vi "WriteGPSRefernceData.vi"(0 "LatitudeRef":string="South", 1 "ExifTool Path":path=path "C:/Windows/System32", 5 "LongitudeRef":string="East", 7 "AltitudeRef":string="Above Sea Level", 9 "filepath":string, 11 "error in (no error)":errorcluster, 12 "wait until completion? (T)":bool=TRUE) -> (4 "standard error":string, 15 "error out":errorcluster)   [LabVIEW 2016]
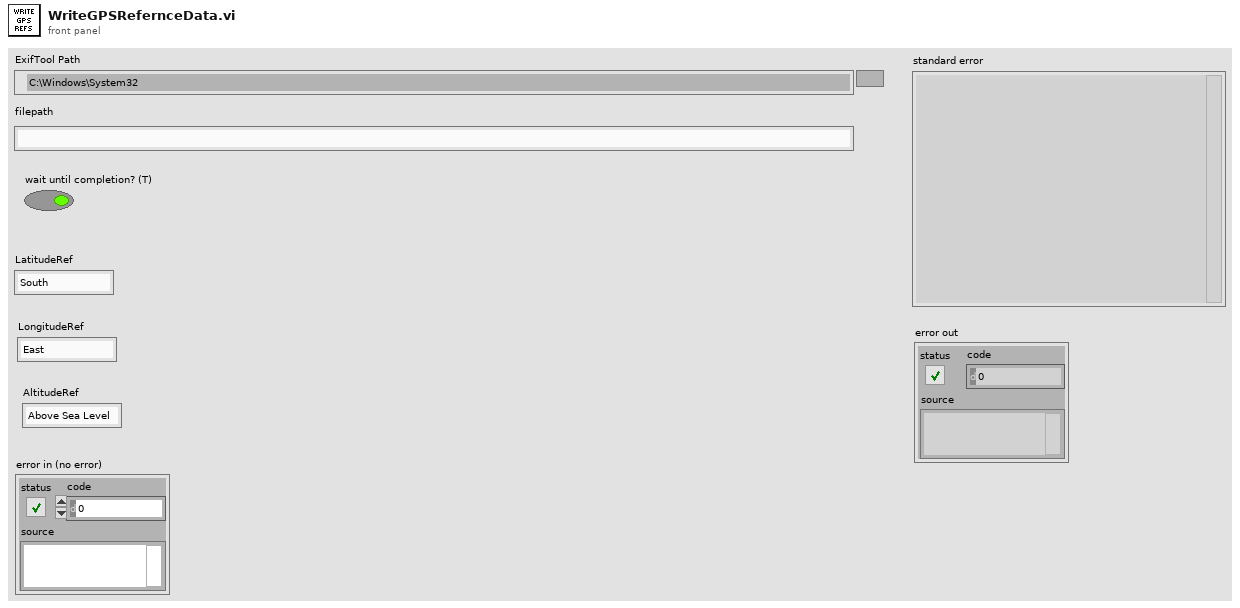
[diagram p1: front panel]
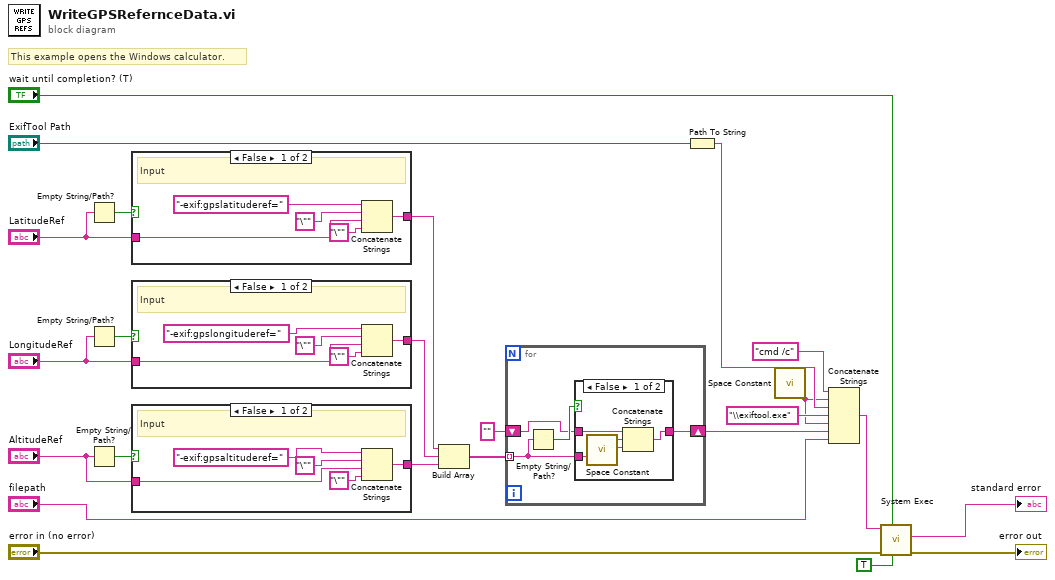
[diagram p0: block diagram]
diagram:
  # "This example opens the Windows calculator."
  n1 = Empty String/Path?(string/path="LatitudeRef") -> (empty?=w18:bool)
  n2 = Empty String/Path?(string/path="LongitudeRef") -> (empty?=w15:bool)
  n3 = Empty String/Path?(string/path="AltitudeRef") -> (empty?=w13:bool)
  n4 = case shown="False" w18 {
    tunnel: "LatitudeRef" -> [w27 _]
    tunnel: [w25 _] -> w12
    frame False {
      # "Input"
      n5 = Concatenate Strings("-exif:gpslatituderef=" ("string"), "\"" ("string"), w27, "\"" ("string")) -> (w25:string)
    }
    frame True {
    }
  }
  n6 = case shown="False" w15 {
    tunnel: "LongitudeRef" -> [w32 _]
    tunnel: [w30 _] -> w11
    frame False {
      # "Input"
      n7 = Concatenate Strings("-exif:gpslongituderef=" ("string"), "\"" ("string"), w32, "\"" ("string")) -> (w30:string)
    }
    frame True {
    }
  }
  n8 = case shown="False" w13 {
    tunnel: "AltitudeRef" -> [w37 _]
    tunnel: [w35 _] -> w10
    frame False {
      # "Input"
      n9 = Concatenate Strings("-exif:gpsaltituderef=" ("string"), "\"" ("string"), w37, "\"" ("string")) -> (w35:string)
    }
    frame True {
    }
  }
  n10 = Build Array(w12, w11, w10) -> (w9:string[])
  n11 = for {
    tunnel: w9 -> [w40] mode=indexing
    shift-right: [w41] -> w7
    shift-left: "" -> [w42]
    n12 = Empty String/Path?(string/path=w40) -> (empty?=w43:bool)
    n13 = case shown="False" w43 {
      tunnel: w42 -> [w47 w48]
      tunnel: [w45 w48] -> w41
      tunnel: w40 -> [w44 _]
      frame False {
        n14 = call <vilib>:"Space Constant.vi"() -> ("String"=w46:string)
        n15 = Concatenate Strings(w47, w44, w46) -> (w45:string)
      }
      frame True {
      }
    }
  }
  n16 = Path To String(path="ExifTool Path") -> (string=w21:string)
  n17 = call <vilib>:"Space Constant.vi"() -> ("String"=w19:string)
  n18 = Concatenate Strings("cmd /c" ("string"), w19, w21, "\\exiftool.exe" ("string"), w19, w7, "filepath") -> (w5:string)
  n19 = call <vilib>:"System Exec.vi"("run minimized? (F)"=TRUE, "wait until completion? (T)"="wait until completion? (T)", "error in (no error)"="error in (no error)", "command line"=w5) -> ("error out"=→"error out":errorcluster, "standard error"=→"standard error":string)  [unwired: 4 in, 2 out]
